vi "Register for Panel Events.vi"(8 "error in (no error)":errorcluster, 9 "Controls to Exclude":refnum<vi>[](array[refnum]), 10 "VI Refnum (Caller)":refnum<vi>) -> (0 "error out":errorcluster, 1 "Stop! Event":refnum<user-event>, 2 "Event Registration Refnum":refnum<event-registration>, 3 "AbstractAutoRegistration out":refnum<class "AutoRegistration.lvclass">)   [LabVIEW 2015, in "AutoRegistration.lvlib" / "AutoRegistration.lvclass"]
uses:
  AutoRegistration.lvclass
  Registration References.ctl
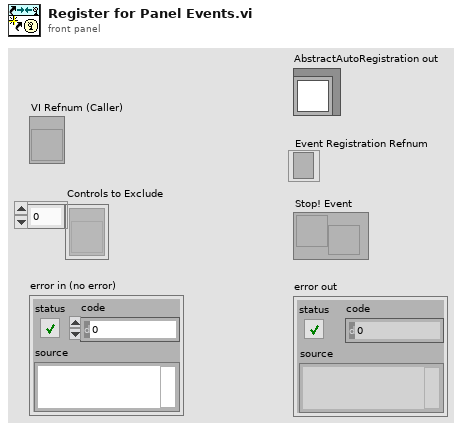
[diagram p1: front panel]
types:
  T1 = typedef "AutoRegistration.lvlib/AutoRegistration.lvclass/Registration References.ctl" = cluster{"Switching Boolean":refnum<vi>[], "Latching Boolean":refnum<vi>[], "I8":refnum<vi>[], "I16":refnum<vi>[], "I32":refnum<vi>[], "I64":refnum<vi>[], "U8":refnum<vi>[], "U16":refnum<vi>[], "U32":refnum<vi>[], "U64":refnum<vi>[], "SGL":refnum<vi>[], "DBL":refnum<vi>[], "EXT":refnum<vi>[], "FXP":refnum<vi>[], "String":refnum<vi>[], "Path":refnum<vi>[], "Timestamp":refnum<vi>[], "Other Controls":refnum<vi>[]}
  T2 = enum32{"Invalid", "Standard", "Closed", "Hidden", "Minimized", "Maximized"}
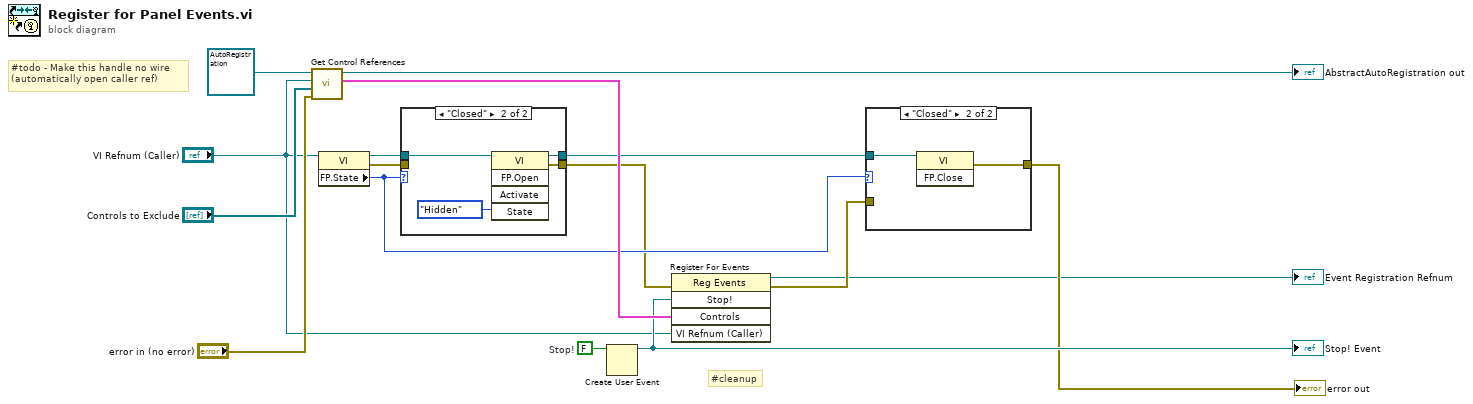
[diagram p0: block diagram]
diagram:
  w13 = FALSE  # Stop!
  # "#cleanup"
  # "#todo - Make this handle no wire\n(automatically open caller ref)"
  n1 = call-dynamic "Get Control References.vi"("error in (no error)"="error in (no error)", "Controls to Exclude"="Controls to Exclude", "VI Refnum"="VI Refnum (Caller)", "AutoRegistration In"=refnum<class "AutoRegistration.lvclass"> refnum ("AbstractAutoRegistration in")) -> ("Controls"=w16:T1, "AutoRegistration Out"=→"AbstractAutoRegistration out":refnum<class "AutoRegistration.lvclass">)  [unwired: 5 in, 1 out]
  n2 = property on="Property Node" class="VI"(reference="VI Refnum (Caller)") -> (reference out=w11:refnum<vi>, error out=w8:errorcluster, "FP.State"=w9:T2)  [unwired: 1 in]
  n3 = case shown="\"Closed\"" w9 {
    tunnel: w11 -> [w18 w21]
    tunnel: [w17 w20] -> w7
    tunnel: [w18 w19] -> w10
    tunnel: w8 -> [w17 _]
    frame Default {
    }
    frame "Closed" {
      n4 = invoke on="Invoke Node" class="VI" method="FP.Open"(reference=w21, "State"=T2."Hidden") -> (reference out=w19:refnum<vi>, error out=w20:errorcluster)  [unwired: 3 in, 3 out]
    }
  }
  n5 = Create User Event(user event datatype=w13) -> (user event=w14:refnum<user-event>)  [unwired: 1 in, 1 out]
  "Stop! Event" <- w14
  n6 = register-events(error in=w7, w14, w16, "VI Refnum (Caller)") -> (reference out=→"Event Registration Refnum":refnum<event-registration>, error out=w6:errorcluster)  [unwired: 1 in]
  n7 = case shown="\"Closed\"" w9 {
    tunnel: w10 -> [_ w24]
    tunnel: w6 -> [_ _]
    tunnel: [_ w23] -> w5
    frame Default {
    }
    frame "Closed" {
      n8 = invoke on="Invoke Node" class="VI" method="FP.Close"(reference=w24) -> (error out=w23:errorcluster)  [unwired: 2 in, 2 out]
    }
  }
  "error out" <- w5
